vi "Komponente aus SPAN Idx.vi"(10 "Component Index":i32=1, 11 "index of element":i32) -> (3 "Komponente:":u16)   [LabVIEW 2020, in "Linearisierung v2.lvlib" / "SpanEinstellungen.lvlib"]
uses:
  SpanEinstellungen.lvlib
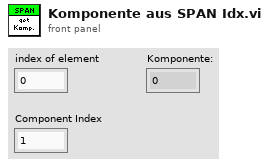
[diagram p1: front panel]
types:
  T1 = cluster{"Komponente:":u16, "Konzentration IST":dbl}[]
  T2 = cluster{"Komponente:":u16, "Konzentration IST":dbl}
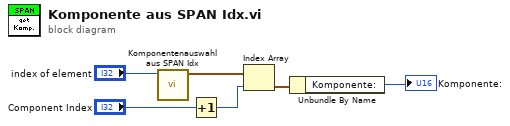
[diagram p0: block diagram]
diagram:
  n1 = call "Komponentenauswahl aus SPAN Idx.vi"("Span Iindex"="index of element") -> ("Komponentenauswahl"=w4:T1)  [unwired: 10 in]
  n2 = Increment(x="Component Index") -> (x+1=w1:i32)
  n3 = Index Array(array=w4, index=w1) -> (element=w5:T2)
  n4 = Unbundle By Name(w5) -> ("Komponente:"=→"Komponente:":u16)
